vi "fgv_PXI-5110_q-data.vi"(7 "cmd":T1, 8 "error in":errorcluster, 11 "wfm":waveform(dbl)={"t0"=timestamp(0 s since 1904-01-01), "dt"=0.0, "Y"=[]}) -> (0 "error out":errorcluster, 3 "queue out":refnum<queue>)   [LabVIEW 2021]
uses:
  ctrl/5110_q.ctl
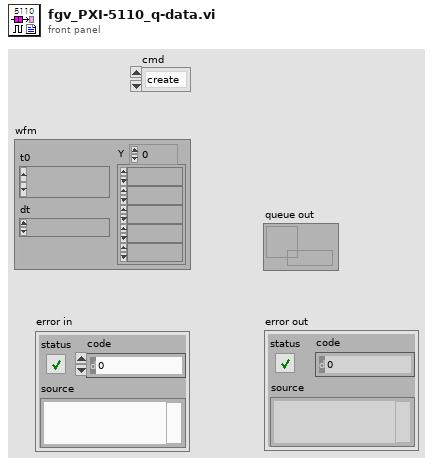
[diagram p1: front panel]
types:
  T1 = typedef "5110_q.ctl" = enum16{"create", "read", "write", "close"}
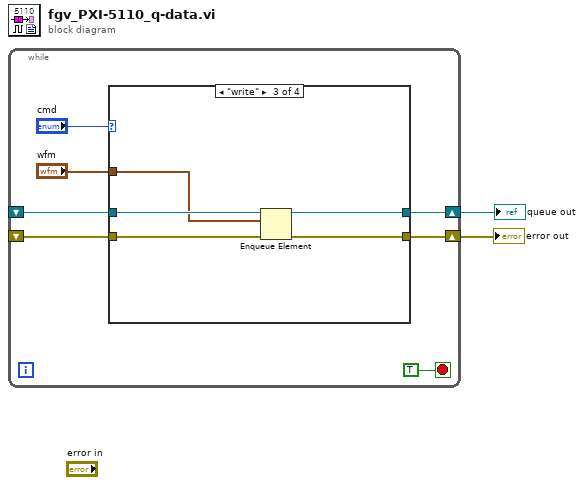
[diagram p0: block diagram]
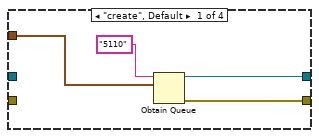
[diagram p2: hidden frame]
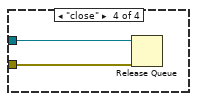
[diagram p4: hidden frame]
diagram:
  n1 = while {
    shift-right: [w7] -> w1
    shift-left: _ -> [w5]
    shift-right: [w6] -> w2
    shift-left: _ -> [w4]
    stop <- TRUE stop-if-true
    n2 = case shown="\"write\"" "cmd" {
      tunnel: [w13 w15 w17 _] -> w7
      tunnel: [w12 w14 w18 _] -> w6
      tunnel: "wfm" -> [w11 _ w16 _]
      tunnel: w5 -> [_ w15 w20 w22]
      tunnel: w4 -> [_ w14 w19 w21]
      frame "create", Default {
        n3 = Obtain Queue(name (unnamed)="5110", element data type=w11) -> (queue out=w13:refnum<queue>, error out=w12:errorcluster)  [unwired: 3 in, 1 out]
      }
      frame "read" {
      }
      frame "write" {
        n4 = Enqueue Element(queue=w20, element=w16, error in (no error)=w19) -> (queue out=w17:refnum<queue>, error out=w18:errorcluster)  [unwired: 1 in, 1 out]
      }
      frame "close" {
        n5 = Release Queue(queue=w22, error in (no error)=w21) -> ()  [unwired: 1 in, 3 out]
      }
    }
  }
  "error out" <- w2
  "queue out" <- w1
